vi "dfd_TF to Lattice ARMA.vi"(9 "section type":T1(ring), 10 "denominator":dbl[](array[numeric]) format="%.2f", 11 "numerator":dbl[](array[numeric]) format="%.2f") -> (0 "fail?":bool, 2 "k [1~M]":dbl[](array[numeric]) format="%.2f", 3 "v [0~M]":dbl[](array[numeric]) format="%.2f")   [LabVIEW 2017, in "NI_DigFilterLicensed.lvlib"]
uses:
  <vilib>/addons/Digital Filter Design/NI_DigFilterLicensed.lvlib
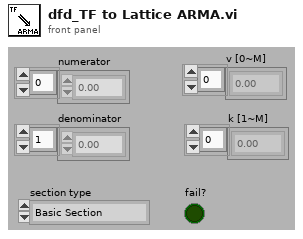
[diagram p1: front panel]
types:
  T1 = enum16{"Basic Section", "One Multiplier Section", "Normalized Section"}
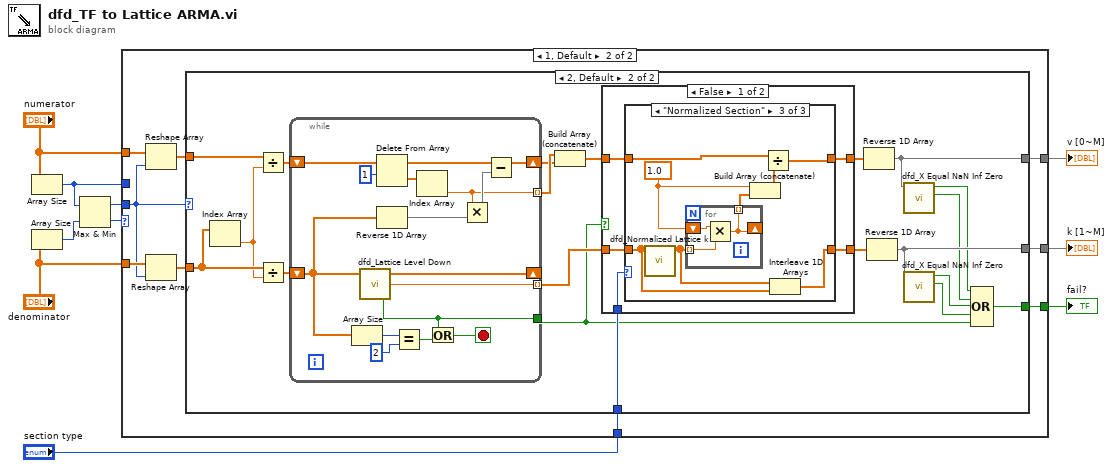
[diagram p0: block diagram]
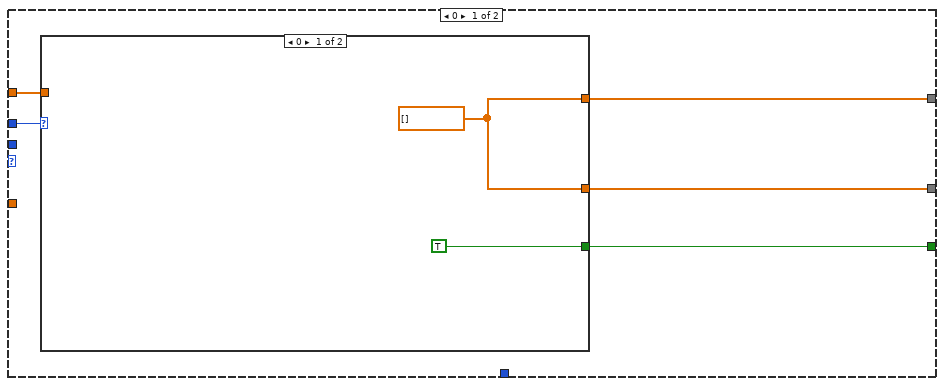
[diagram p2: hidden frame]
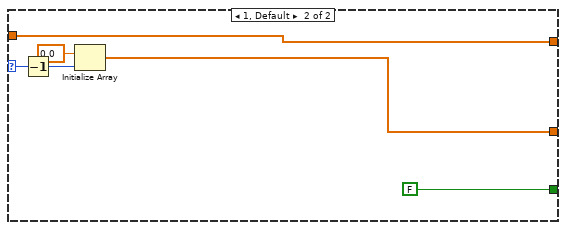
[diagram p3: hidden frame]
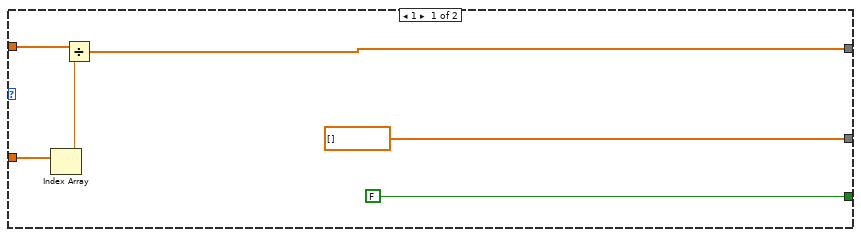
[diagram p4: hidden frame]
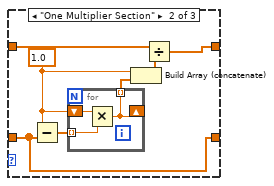
[diagram p6: hidden frame]
diagram:
  n1 = Array Size(array="numerator") -> (size(s)=w8:i32)
  n2 = Array Size(array="denominator") -> (size(s)=w10:i32)
  n3 = Max & Min(x=w8, y=w10) -> (max(x,y)=w7:i32, min(x,y)=w5:i32)
  n4 = case shown="1, Default" w5 {
    tunnel: "denominator" -> [_ w32]
    tunnel: "numerator" -> [w11 w31]
    tunnel: [w12 w24] -> w2
    tunnel: [w13 w25] -> w3
    tunnel: w7 -> [_ w29]
    tunnel: [w15 w26] -> w1
    tunnel: w8 -> [w14 _]
    tunnel: "section type" -> [_ w27]
    frame 0 {
      n5 = case shown="0" w14 {
        selector: w14 -> [_ w20]
        tunnel: [w17 w22] -> w13
        tunnel: [TRUE ("fail?") FALSE ("fail?")] -> w15
        tunnel: [w17 w18] -> w12
        tunnel: w11 -> [_ w22]
        frame 0 {
          w17 = dbl[] [] ("coefficients out")
        }
        frame 1, Default {
          n6 = Decrement(x=w20) -> (x-1=w21:i32)
          n7 = Initialize Array(0.0 ("element"), w21) -> (w18:dbl[])
        }
      }
    }
    frame 1, Default {
      n8 = Reshape Array(w31, w29) -> (w30:dbl[])
      n9 = Reshape Array(w32, w29) -> (w28:dbl[])
      n10 = case shown="2, Default" w29 {
        tunnel: w28 -> [w36 w56]
        tunnel: w30 -> [w38 w58]
        tunnel: [FALSE w45] -> w26
        tunnel: w27 -> [_ w50]
        tunnel: [w34 w43] -> w25
        tunnel: [dbl[] [] ("coefficients out") w44] -> w24
        frame 1 {
          n11 = Index Array(array=w36) -> (element=w37:dbl)  [unwired: 1 in]
          n12 = Divide(x=w38, y=w37) -> (x/y=w34:dbl[])
        }
        frame 2, Default {
          n13 = Index Array(array=w56) -> (element=w55:dbl)  [unwired: 1 in]
          n14 = Divide(x=w58, y=w55) -> (x/y=w57:dbl[])
          n15 = Divide(x=w56, y=w55) -> (x/y=w54:dbl[])
          n16 = while {
            shift-right: [w98] -> w52
            shift-left: w57 -> [w102]
            tunnel: [w96] -> w53 mode=indexing
            shift-right: [w94] -> _
            shift-left: w54 -> [w92]
            tunnel: [w93] -> w49 mode=indexing
            tunnel: [w87] -> w46
            stop <- w88 stop-if-true
            n17 = Array Size(array=w92) -> (size(s)=w91:i32)
            n18 = call <vilib>:"dfd_Lattice Level Down.vi"("Bm(z)"=w92) -> ("Bm-1(z)"=w94:dbl[], "km"=w93:dbl, "fail?"=w87:bool)
            n19 = Delete From Array(array=w102, length=1) -> (deleted portion=w100:dbl[], array with subset deleted=w99:dbl[])  [unwired: 1 in]
            n20 = Reverse 1D Array(array=w92) -> (reversed array=w95:dbl[])
            n21 = Equal?(x=w91, y=2) -> (x = y?=w89:bool)
            n22 = Index Array(array=w100) -> (element=w96:dbl)  [unwired: 1 in]
            n23 = Or(x=w87, y=w89) -> (x .or. y?=w88:bool)
            n24 = Multiply(x=w96, y=w95) -> (x*y=w97:dbl[])
            n25 = Subtract(x=w99, y=w97) -> (x-y=w98:dbl[])
          }
          n26 = Build Array (concatenate)(w53, w52) -> (w51:dbl[])
          n27 = case shown="False" w46 {
            tunnel: w51 -> [w63 _]
            tunnel: w49 -> [w62 _]
            tunnel: w50 -> [w61 _]
            tunnel: [w60 _] -> w47
            tunnel: [w59 _] -> w48
            frame False {
              n28 = case shown="\"Normalized Section\"" w61 {
                tunnel: w63 -> [w65 w72 w83]
                tunnel: w62 -> [w64 w66 w77]
                tunnel: [w65 w71 w82] -> w60
                tunnel: [w64 w66 w78] -> w59
                frame "Basic Section", Default {
                }
                frame "One Multiplier Section" {
                  w68 = 1.0
                  n29 = Subtract(x=w68, y=w66) -> (x-y=w70:dbl[])
                  n30 = for {
                    tunnel: [w73] -> w69 mode=indexing
                    tunnel: w70 -> [w74] mode=indexing
                    shift-right: [w73] -> _
                    shift-left: w68 -> [w75]
                    n31 = Multiply(x=w75, y=w74) -> (x*y=w73:dbl)
                  }
                  n32 = Build Array (concatenate)(w68, w69) -> (w67:dbl[])
                  n33 = Divide(x=w72, y=w67) -> (x/y=w71:dbl[])
                }
                frame "Normalized Section" {
                  w80 = 1.0
                  n34 = call <vilib>:"dfd_Normalized Lattice k.vi"("k"=w77) -> ("^k"=w76:dbl[])  [unwired: 10 out]
                  n35 = for {
                    tunnel: [w84] -> w81 mode=indexing
                    tunnel: w76 -> [w85] mode=indexing
                    shift-right: [w84] -> _
                    shift-left: w80 -> [w86]
                    n36 = Multiply(x=w86, y=w85) -> (x*y=w84:dbl)
                  }
                  n37 = Build Array (concatenate)(w80, w81) -> (w79:dbl[])
                  n38 = Divide(x=w83, y=w79) -> (x/y=w82:dbl[])
                  n39 = Interleave 1D Arrays(w76, w77) -> (w78:dbl[])
                }
              }
            }
            frame True {
            }
          }
          n40 = Reverse 1D Array(array=w47) -> (reversed array=w43:dbl[])
          n41 = Reverse 1D Array(array=w48) -> (reversed array=w44:dbl[])
          n42 = call <vilib>:"dfd_X Equal NaN Inf Zero.vi"("roots"=w43) -> ("contain Inf ?"=w41:bool, "contain NaN ?"=w42:bool)  [unwired: 9 out]
          n43 = call <vilib>:"dfd_X Equal NaN Inf Zero.vi"("roots"=w44) -> ("contain Inf ?"=w39:bool, "contain NaN ?"=w40:bool)  [unwired: 9 out]
          n44 = Compound Arithmetic op=OR(w42, w41, w40, w39, w46) -> (w45:bool)
        }
      }
    }
  }
  "k [1~M]" <- w2
  "v [0~M]" <- w3
  "fail?" <- w1
